vi "construct.vi"(6 "tablecloth_type":T1 items=["Type 1", "Type 2"], 8 "error in (no error)":errorcluster, 9 "cost":dbl, 10 "id":u32) -> (0 "error out":errorcluster, 3 "table out":refnum<class "Table.lvclass">)   [LabVIEW 2021, in "Table.lvclass"]
uses:
  Table.lvclass
  TableclothType.ctl
  Table.lvclass/Table.ctl
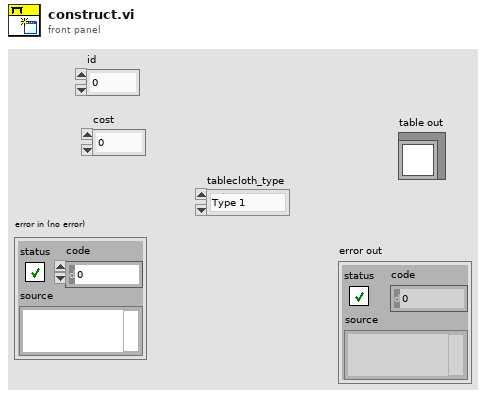
[diagram p1: front panel]
types:
  T1 = typedef "Table.lvclass/TableclothType.ctl" = u16
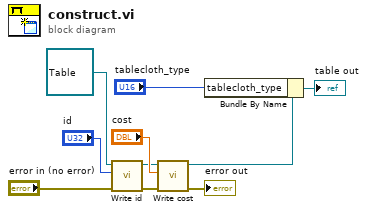
[diagram p0: block diagram]
diagram:
  n1 = call-dynamic "Write id.vi"("error in (no error)"="error in (no error)", "id"="id", "Furniture in"=refnum<class "Table.lvclass"> refnum ("Table.lvclass")) -> ("error out"=w8:errorcluster, "Furniture out"=w5:refnum<class "Table.lvclass">)  [unwired: 7 in]
  n2 = call-dynamic "Write cost.vi"("error in (no error)"=w8, "price"="cost", "Furniture in"=w5) -> ("error out"=→"error out":errorcluster, "Furniture out"=w3:refnum<class "Table.lvclass">)  [unwired: 7 in]
  n3 = Bundle By Name(cluster=w3, "tablecloth_type"="tablecloth_type") -> (→"table out":refnum<class "Table.lvclass">)
